vi "Get Report Nb_Octet.vi"(8 "error in (no error)":errorcluster caption="entrée d'erreur (pas d'erreur)", 11 "Nodon_Send_Command_UART en entrée":refnum<class "Nodon_Send_Command_UART.lvclass">) -> (0 "error out":errorcluster caption="sortie d'erreur", 2 "Report Nb_Octet":u16, 3 "Nodon_Send_Command_UART en sortie":refnum<class "Nodon_Send_Command_UART.lvclass">)   [LabVIEW 2020, in "Library Test.lvlib" / "Nodon_Send_Command_UART.lvclass"]
uses:
  Nodon_Send_Command_UART.lvclass
  Nodon_Send_Command_UART.lvclass/Nodon_Send_Command_UART.ctl
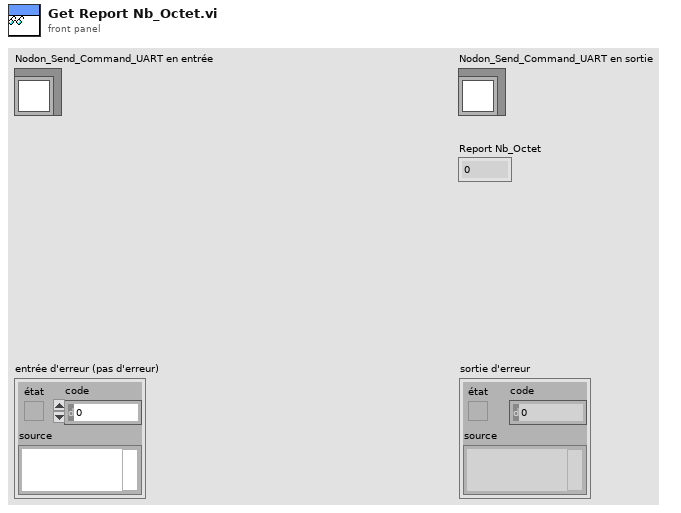
[diagram p1: front panel]
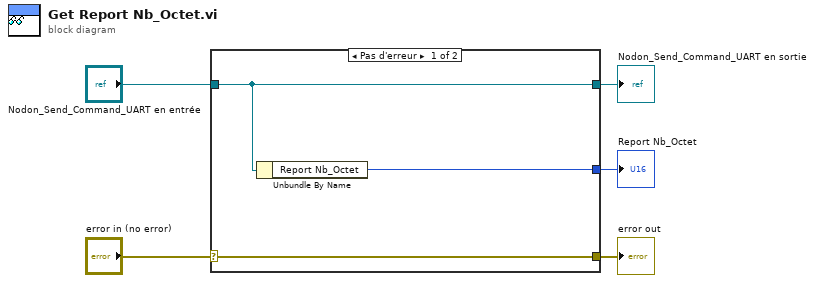
[diagram p0: block diagram]
diagram:
  n1 = case shown="Pas d'erreur" "error in (no error)" {
    selector: "error in (no error)" -> [w8 w9]
    tunnel: [w8 w9] -> w4
    tunnel: [w7 w10] -> w2
    tunnel: "Nodon_Send_Command_UART en entrée" -> [w7 w10]
    tunnel: [w6 _] -> w1
    frame No Error {
      n2 = Unbundle By Name(w7) -> ("Report Nb_Octet"=w6:u16)
    }
    frame Error {
    }
  }
  "error out" <- w4
  "Nodon_Send_Command_UART en sortie" <- w2
  "Report Nb_Octet" <- w1
